vi "DAQ Abort.vi"(7 "error in":errorcluster) -> (0 "error out":errorcluster)   [LabVIEW 2011]
uses:
  Functional Global Data/Globals.ctl
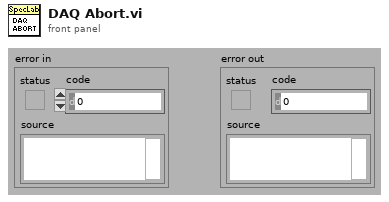
[diagram p1: front panel]
types:
  T1 = typedef "Globals.ctl" = enum16{"Initialize", "Get DAQ Params", "Get Data Display Params", "Set DAQ Params", "Set Data Display Params"}
  T2 = typedef "Data Acquisition Parameters.ctl" = cluster{"Experiment Type":T3, "Experiment Name":string, "Operator Name":string, "Notes":string, "TDMS File Path":path, "Data Acquisition State":bool, "PID Voltage Sweep":T4, "MFC Challenge Profile - Heaviside Step":T5, "MFC Challenge Profile":T6, "MFC Challenge Profile - Staircase":T7}
  T3 = typedef "DAQ Type.ctl" = enum16{"PID Sample", "PID with PS Challenge", "PID with MFC Challenge", "Multimeter Sample", "Multimeter with MFC Challenge"}
  T4 = typedef "PID Voltage Seep Settings.ctl" = cluster{"Voltage Step (V)":dbl, "Voltage Range (V)":cluster{u16, u16}, "Time Step (s)":dbl, "Voltage Step Direction":enum16{"High 2 Low", "Low 2 High"}}
  T5 = typedef "MFC Challenge Profile - Heaviside Step.ctl" = cluster{"Valve Open Duration":u16, "MFC Flow Rate":dbl, "Valve Open Repeats":u16, "Valve Open Start":u16}
  T6 = typedef "MFC Challen Profile Type.ctl" = enum16{"Heaviside", "Staircase"}
  T7 = typedef "MFC Challenge Profile - Staircase.ctl" = cluster{"Step Time Duration":u16, "Step Flow Rate":dbl, "Steps":u16, "Valve Open Start":u16, "Recovery":bool, "Repeats":u16}
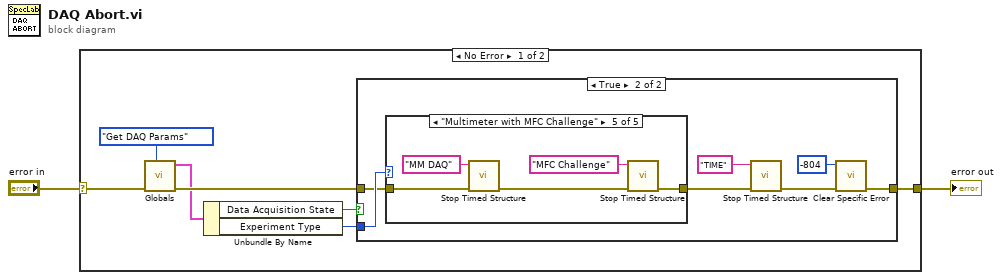
[diagram p0: block diagram]
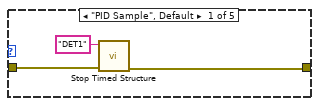
[diagram p3: hidden frame]
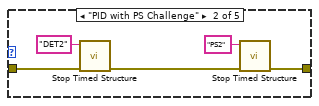
[diagram p4: hidden frame]
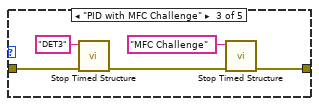
[diagram p5: hidden frame]
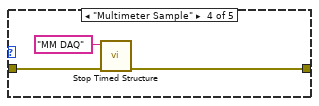
[diagram p6: hidden frame]
diagram:
  n1 = case shown="No Error" "error in" {
    selector: "error in" -> [w7 w39]
    tunnel: [w6 w39] -> w1
    frame No Error {
      n2 = call "Globals.vi"("action"=Globals."Get DAQ Params", "error in"=w7) -> ("error out"=w8:errorcluster, "Data Acquisition"=w5:T2)  [unwired: 7 in, 1 out]
      n3 = Unbundle By Name(w5) -> ("Data Acquisition State"=w3:bool, "Experiment Type"=w4:T3)
      n4 = case shown="True" w3 {
        tunnel: [w10 w16] -> w6
        tunnel: w8 -> [w10 w14]
        tunnel: w4 -> [_ w15]
        frame False {
        }
        frame True {
          n5 = case shown="\"Multimeter with MFC Challenge\"" w15 {
            tunnel: [w18 w23 w26 w31 w34] -> w12
            tunnel: w14 -> [w19 w22 w29 w32 w37]
            frame "PID Sample", Default {
              n6 = call <vilib>:"Stop Timed Structure.vi"("error in (no error)"=w19, "name"="DET1") -> ("error out"=w18:errorcluster)  [unwired: 9 in]
            }
            frame "PID with PS Challenge" {
              n7 = call <vilib>:"Stop Timed Structure.vi"("error in (no error)"=w22, "name"="DET2") -> ("error out"=w21:errorcluster)  [unwired: 9 in]
              n8 = call <vilib>:"Stop Timed Structure.vi"("error in (no error)"=w21, "name"="PS2") -> ("error out"=w23:errorcluster)  [unwired: 9 in]
            }
            frame "PID with MFC Challenge" {
              n9 = call <vilib>:"Stop Timed Structure.vi"("error in (no error)"=w29, "name"="DET3") -> ("error out"=w27:errorcluster)  [unwired: 9 in]
              n10 = call <vilib>:"Stop Timed Structure.vi"("error in (no error)"=w27, "name"="MFC Challenge") -> ("error out"=w26:errorcluster)  [unwired: 9 in]
            }
            frame "Multimeter Sample" {
              n11 = call <vilib>:"Stop Timed Structure.vi"("error in (no error)"=w32, "name"="MM DAQ") -> ("error out"=w31:errorcluster)  [unwired: 9 in]
            }
            frame "Multimeter with MFC Challenge" {
              n12 = call <vilib>:"Stop Timed Structure.vi"("error in (no error)"=w37, "name"="MM DAQ") -> ("error out"=w35:errorcluster)  [unwired: 9 in]
              n13 = call <vilib>:"Stop Timed Structure.vi"("error in (no error)"=w35, "name"="MFC Challenge") -> ("error out"=w34:errorcluster)  [unwired: 9 in]
            }
          }
          n14 = call <vilib>:"Stop Timed Structure.vi"("error in (no error)"=w12, "name"="TIME") -> ("error out"=w11:errorcluster)  [unwired: 9 in]
          n15 = call "Clear Specific Error.vi"("error in"=w11, "code"=-804 ("Code")) -> ("error out"=w16:errorcluster)  [unwired: 5 in]
        }
      }
    }
    frame Error {
    }
  }
  "error out" <- w1
